vi "7-2 hp34401A generatore di funzioni sol.vi"(0 "N":i32=10, 2 "Limite":dbl format="%.2f", 3 "stop":bool) -> (1 "Tipo di strumento":string, 4 "error out":bool, 5 "Sopra il limite":bool, 6 "vet-dati":dbl[](array[numeric]) format="%.2f", 7 "Max":dbl format="%.2f", 8 "Med":dbl format="%.2f")   [LabVIEW 2012]
doc: "© Copyright M. Ferrari- M. Corti 2003-2005\n Repeated Gpib Measurements"
uses:
  <vilib>/Analysis/baseanly.llb/Mean (DBL).vi
  <vilib>/Analysis/NI_AALBase.lvlib
panel:
  out "error code out":i16=-1
  out "Grafico":dbl(graph)
  in  "addr":string="4"
  # "4. IDENTIFICAZIONE dello STRUMENTO, CONFIGURAZIONE, MISURE RIPETUTE, RAPPRESENTAZIONE dei    \n    VALORI in TEMPO REALE, ANALISI\n    Realizzare un VI che svolga le seguenti funzioni:\n   - richiede l'identificazione dello strumento Hewlett-Packard collegato al bus IEEE 488 e ne visualizza il tipo (es. 34401A) \n   - configura lo strumento per una misura di tensione DC su un range di 1 volt, con una risoluzione di 0.1 mV\n   - effettua un numero N di misure (impostabile da pannello) con un ritardo di 0,5 sec l'una dall'altra, gestendo eventuali \n     errori sull'interfaccia e segnalandone la presenza\n   - visualizza i valori acquisiti su di un grafico in tempo reale e, al termine, li memorizza in un vettore \n   - ricava il valore massimo, il valor medio e verifica (con visualizzazione tramite un indicatore booleano) se almeno uno, tra \n     i valori misurati, supera un valore limite selezionabile da pannello\n   - apportare alla soluzione proposta le modifiche eventualmente necessarie perch sia possibile concludere la misura  tramite \n     l'azione, da pannello, su un pulsante di STOP o in caso di errore."
  # "(n¡ misure)"
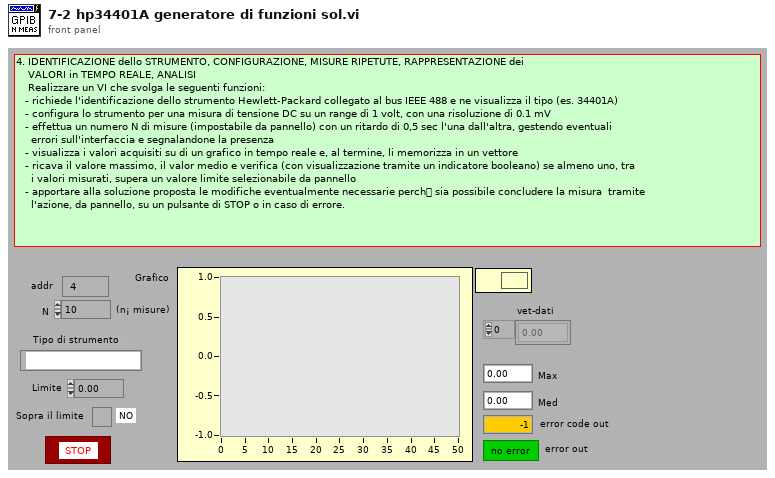
[diagram p1: front panel]
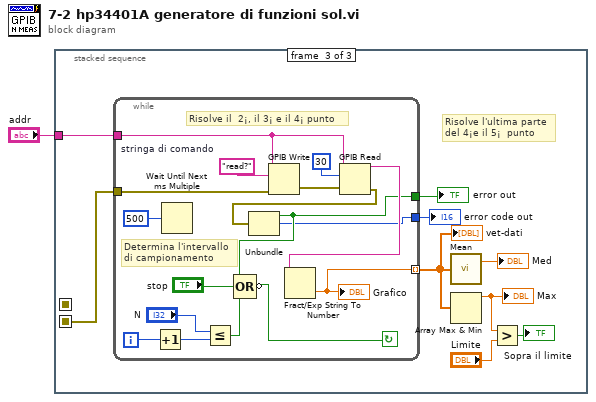
[diagram p0: block diagram]
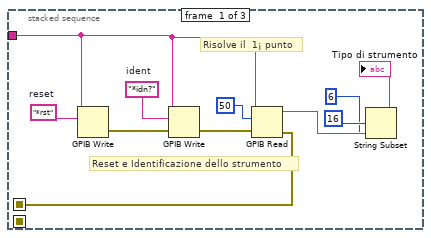
[diagram p2: hidden frame]
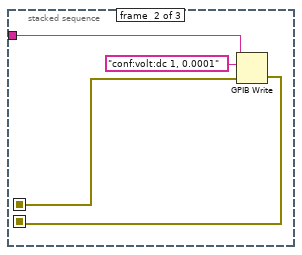
[diagram p3: hidden frame]
diagram:
  n1 = stacked-sequence {
    seq-local: [w4 _ _] -> [_ w14 _]
    seq-local: [_ w13 _] -> [_ _ w17]
    tunnel: "addr" -> [w3 w15 w21]
    frame #0 {
      w10 = "*rst"  # reset
      w8 = "*idn?"  # ident
      # "Risolve il  1¡ punto"
      # "Reset e Identificazione dello strumento"
      n2 = GPIB Write(0:w3, 1:w10) -> (6:w7:errorcluster)  [unwired: 3 in, 1 out]
      n3 = GPIB Write(0:w3, 1:w8, 3:w7) -> (6:w6:errorcluster)  [unwired: 2 in, 1 out]
      n4 = GPIB Read(0:w3, 1:50 ("n° byte"), 3:w6) -> (5:w5:string, 7:w4:errorcluster)  [unwired: 2 in, 1 out]
      n5 = String Subset(string=w5, offset (0)=16, length (rest)=6) -> (substring=→"Tipo di strumento":string)
    }
    frame #1 {
      n6 = GPIB Write(0:w15, 1:"conf:volt:dc 1, 0.0001" ("data"), 3:w14) -> (6:w13:errorcluster)  [unwired: 2 in, 1 out]
    }
    frame #2 {
      # "Risolve l'ultima parte\ndel 4¡e il 5¡  punto"
      n7 = while {
        tunnel: w21 -> [w38]
        tunnel: w17 -> [w29]
        tunnel: [w37] -> w20 mode=indexing
        tunnel: [w27] -> w19
        tunnel: [w26] -> w18
        i -> [w35]
        stop <- w30 continue-if-true
        w42 = "read?"  # stringa di comando
        # "Risolve il  2¡, il 3¡ e il 4¡ punto"
        # "Determina l'intervallo\ndi campionamento"
        n8 = Increment(x=w35) -> (x+1=w33:i32)
        n9 = Wait Until Next ms Multiple(millisecond multiple=u32 500) -> ()  [unwired: 1 out]
        n10 = Less Or Equal?(x="N", y=w33) -> (x <= y?=w31:bool)
        n11 = GPIB Write(0:w38, 1:w42, 3:w29) -> (6:w41:errorcluster)  [unwired: 2 in, 1 out]
        n12 = GPIB Read(0:w38, 1:30, 3:w41) -> (5:w39:string, 7:w28:errorcluster)  [unwired: 2 in, 1 out]
        n13 = Unbundle(w28) -> ("status"=w27:bool, "code"=w26:i32)  [unwired: 1 out]
        n14 = Compound Arithmetic op=OR(w27, "stop", w31) -> (invert w30:bool)
        n15 = Fract/Exp String To Number(string=w39) -> (number=w37:dbl)  [unwired: 3 in, 1 out]
        "Grafico" <- w37
      }
      "vet-dati" <- w20
      "error out" <- w19
      "error code out" <- w18
      n16 = call-poly <vilib>:"Mean.vi"("X"=w20) -> ("mean"=→"Med":dbl)  [unwired: 1 out]
      n17 = Array Max & Min(array=w20) -> (max value=w24:dbl)  [unwired: 3 out]
      "Max" <- w24
      n18 = Greater?(x=w24, y="Limite") -> (0:→"Sopra il limite":bool)
    }
  }
